vi "SR430.Reset.vi"(0 "i ref in":refnum<vi>, 5 "error in (no error)":errorcluster) -> (14 "i ref out":refnum<vi>, 19 "error out":errorcluster)   [LabVIEW 2014, in "SR430.lvlib"]
doc: "This is a Method that should be by changed by each daughter to class to implement a proper reset function."
uses:
  SR430.lvlib
  CS_Core/CSSystem/CoreDefs/CoreDefs.error_type.ctl
  instr.lib/SR430/SR430Driver.lvlib
  CS_Core/CSSystem/CoreLib/CoreLib.lvlib
  CS_Core/CSApplicationBaseClasses/DeviceBase/DeviceBase.lvlib
  CS_Core/CSApplicationBaseClasses/MCSBase/MCSBase.lvlib
  CSlibraries/UtilityLib/UtilityLib.lvlib
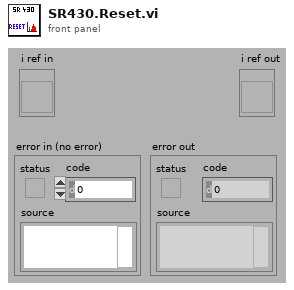
[diagram p1: front panel]
types:
  T1 = typedef "CoreDefs.error_type.ctl" = enum16{"no error", "can't load process", "can't unload process", "process does not exist", "can't install process", "can't remove process", "unknown function", "time out", "can't execute function", "duplicate queue name", "super not found", "caller queue invalid", "can't ping process", "unknown error", "VISA Error", "VISA timeout", "GPIB timeout", "GPIB error", "communication error", "data type mismatch", "can't read data from OPC server", "can't write data to OPC server", "OET error", "function not implemented", "process already exists", "invalid Shared Variable name", "error writing Shared Variable", "error reading Shared Variable", "invalid client name", "corrupt database", "unknown class", "call not authorized", "parameter out of range", "OET timeout: can't get data to modify", "invalid queue name", "requested operation incompatible with current state", "event undefined", "event disabled", "state undefined", "caller is not a friend", "EventBuilder: bad eventID", "EventBuilder: no DAQ devices", "a thread must not stop itself", "UNUSED ELEMENT4", "DiscArchiver: eventData incomplete", "DiscArchiver: eventData does not belong to run", "DiscArchiver: can't open file", "DiscArchiver: can't write to file", "DiscArchiver: available disc space low", "can't acquire semaphore", "error reading data from database", "notifier object is not existing", "can't register process", "can't unregister process", "illegal event type", "object disabled", "object already exists", "can't change state", "Instrument not found", "no connection to remote node", "invalid reference", "N/A", "UNUSED ELEMENT 1", "element not found", "illegal TCP/IP connection detected", "object does not exist", "invalid access ID", "unknown CS system", "invalid privilige", "unsupported data type", "unsupported server type", "IO server already exists", "Shared Variable already exists"}
  T2 = typedef "SR430Driver.lvlib/SR430_VISA Control.ctl" = cluster{"VISA resource name":refnum<visa-resource-name>}
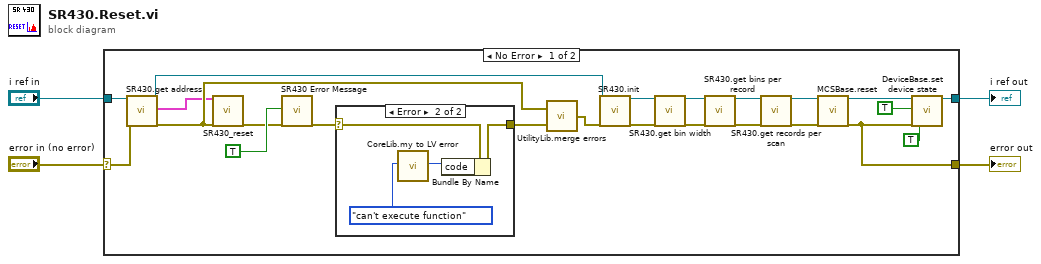
[diagram p0: block diagram]
diagram:
  n1 = case shown="No Error" "error in (no error)" {
    selector: "error in (no error)" -> [w18 w33]
    tunnel: "i ref in" -> [w27 w34]
    tunnel: [w5 w33] -> w3
    tunnel: [w17 w34] -> w2
    frame No Error {
      n2 = call "SR430.get address.vi"("i ref in"=w27, "error in (no error)"=w18) -> ("i ref out"=w24:refnum<vi>, "address"=w25:T2, "error out"=w26:errorcluster)  [unwired: 15 in]
      n3 = call "SR430_reset.vi"("address"=w25, "error in (no error)"=w26) -> ("error out"=w20:errorcluster)  [unwired: 16 in, 1 out]
      n4 = call "SR430 Error Message.vi"("addMessageToSource"=TRUE ("add message to source"), "error in (no error)"=w20) -> ("error out"=w22:errorcluster)  [unwired: 14 in, 3 out]
      n5 = case shown="Error" w22 {
        selector: w22 -> [w28 w31]
        tunnel: [w28 w32] -> w19
        frame No Error {
        }
        frame Error {
          n6 = call "CoreLib.my to LV error.vi"("ErrorTypes"=CoreDefs.error_type."can't execute function") -> ("LV error code"=w30:i32)  [unwired: 17 in, 1 out]
          n7 = Bundle By Name(cluster=w31, "code"=w30) -> (w32:errorcluster)
        }
      }
      n8 = call "UtilityLib.merge errors.vi"("error2 (no error)"=w19, "error1 (no error)"=w26) -> ("error out"=w23:errorcluster)
      n9 = call "SR430.init.vi"("i ref in"=w24, "error in (no error)"=w23) -> ("i ref out"=w14:refnum<vi>, "error out"=w9:errorcluster)  [unwired: 16 in]
      n10 = call "SR430.get bin width.vi"("i ref in"=w14, "error in (no error)"=w9) -> ("i ref out"=w13:refnum<vi>, "error out"=w11:errorcluster)  [unwired: 15 in, 1 out]
      n11 = call "SR430.get bins per record.vi"("i ref in"=w13, "error in (no error)"=w11) -> ("i ref out"=w12:refnum<vi>, "error out"=w10:errorcluster)  [unwired: 15 in, 1 out]
      n12 = call "SR430.get records per scan.vi"("i ref in"=w12, "error in (no error)"=w10) -> ("i ref out"=w7:refnum<vi>, "error out"=w8:errorcluster)  [unwired: 15 in, 1 out]
      n13 = call "MCSBase.reset.vi"("i ref in"=w7, "error in (no error)"=w8) -> ("i ref out"=w6:refnum<vi>, "error out"=w5:errorcluster)  [unwired: 16 in]
      n14 = call "DeviceBase.set device state.vi"("i ref in"=w6, "implicit"=TRUE, "error in (no error)"=w5, "mayResetError (FALSE)"=TRUE) -> ("i ref out"=w17:refnum<vi>)  [unwired: 13 in, 2 out]
    }
    frame Error {
    }
  }
  "error out" <- w3
  "i ref out" <- w2
